vi "testAddStatesToQueueInlining.vi"(8 "error in (no error)":errorcluster, 11 "testStateMachineUtilities in":refnum<class "testStateMachineUtilities.lvclass">) -> (0 "error out":errorcluster, 3 "testStateMachineUtilities out":refnum<class "testStateMachineUtilities.lvclass">)   [LabVIEW 2013, in "testStateMachineUtilities.lvclass"]
uses:
  testStateMachineUtilities.lvclass
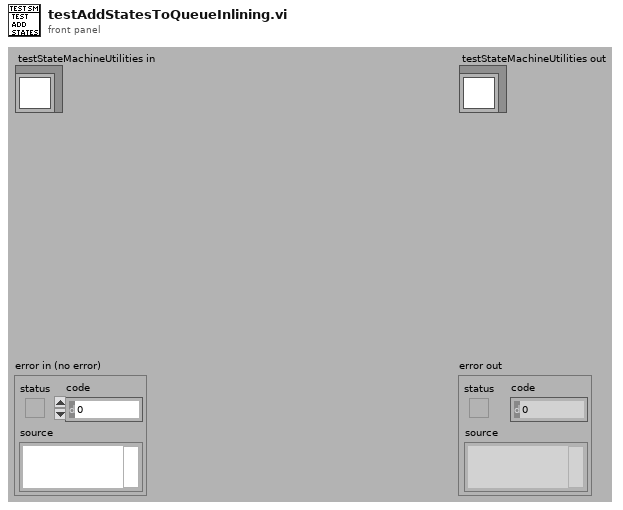
[diagram p1: front panel]
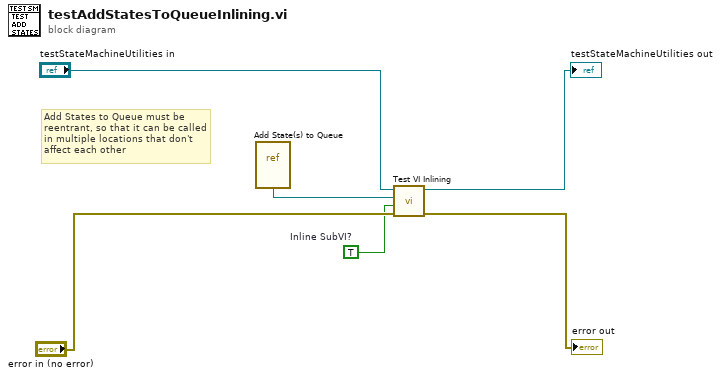
[diagram p0: block diagram]
diagram:
  w1 = TRUE  # Inline SubVI?
  # "Add States to Queue must be reentrant, so that it can be called in multiple locations that don't affect each other"
  n1 = vi-ref "Add State(s) to Queue.vi"() -> (w3:refnum<vi>)
  n2 = call "Test VI Inlining.vi"("error in (no error)"="error in (no error)", "Inline SubVI?"=w1, "VI Refnum"=w3, "testStateMachineUtilities in"="testStateMachineUtilities in") -> ("error out"=→"error out":errorcluster, "testStateMachineUtilities out"=→"testStateMachineUtilities out":refnum<class "testStateMachineUtilities.lvclass">)  [unwired: 6 in]
